vi "Lectura_TDMS.vi"() -> ()   [LabVIEW 2016]
panel:
  out "Waveform Graph 3":waveform(dbl)[](graph)
  out "Waveform Graph 2":waveform(dbl)[](graph)
  out "Waveform Graph":waveform(dbl)[](graph)
  in  "file path":path
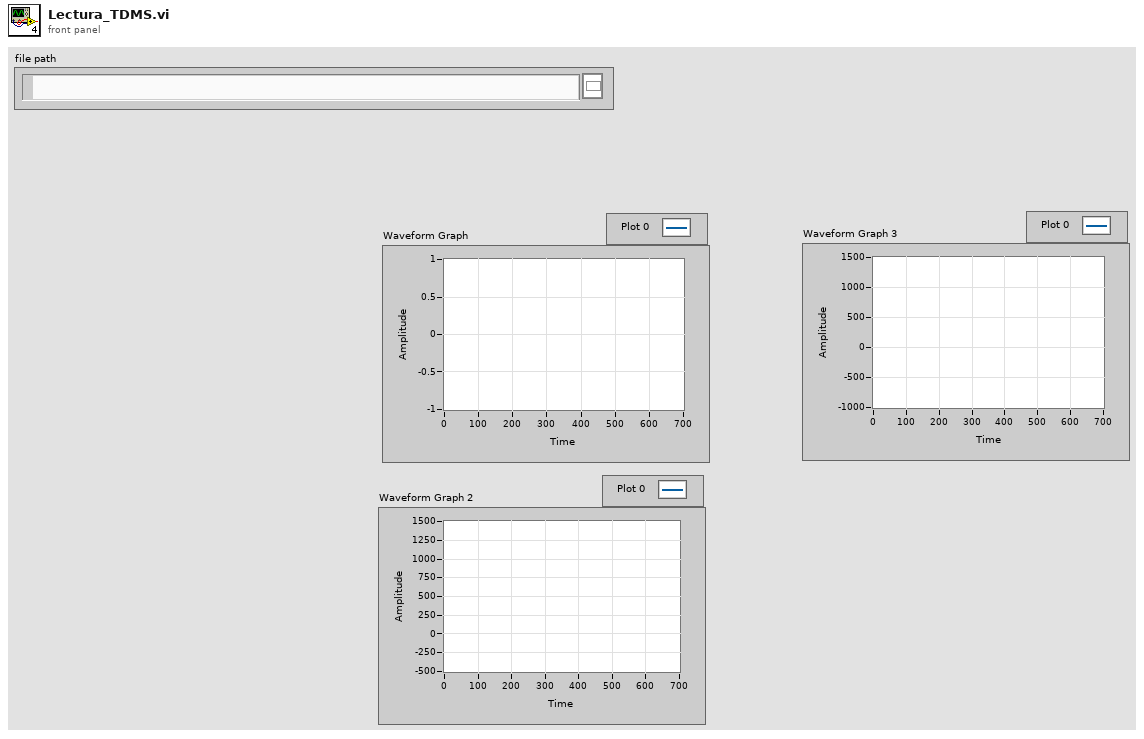
[diagram p1: front panel]
types:
  T1 = enum16{"open", "open or create", "create or replace", "create", "open (read-only)"}
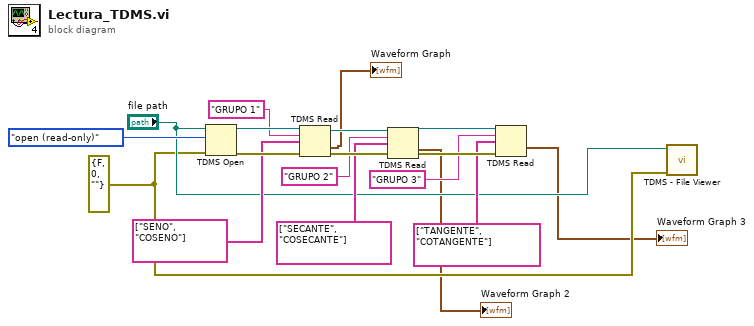
[diagram p0: block diagram]
diagram:
  w4 = errorcluster {"status"=FALSE, "code"=0, "source"=""} ("error in (no error)")
  n1 = TDMS Open(8:w4, 10:T1."open (read-only)" ("operation (0:open)"), 11:"file path") -> (0:w16:errorcluster, 3:w17:refnum<k34>)  [unwired: 4 in]
  n2 = TDMS Read(0:w17, 5:"GRUPO 1" ("group name in (Untitled)"), 7:string[] ["SENO", "COSENO"] ("channel name(s) in (Untitled)"), 11:w16) -> (4:w13:refnum<k34>, 10:→"Waveform Graph":waveform(dbl)[], 15:w12:errorcluster)  [unwired: 4 in, 3 out]
  n3 = TDMS Read(0:w13, 5:"GRUPO 2" ("group name in (Untitled)"), 7:string[] ["SECANTE", "COSECANTE"] ("channel name(s) in (Untitled)"), 11:w12) -> (4:w9:refnum<k34>, 10:→"Waveform Graph 2":waveform(dbl)[], 15:w8:errorcluster)  [unwired: 4 in, 3 out]
  n4 = TDMS Read(0:w9, 5:"GRUPO 3" ("group name in (Untitled)"), 7:string[] ["TANGENTE", "COTANGENTE"] ("channel name(s) in (Untitled)"), 11:w8) -> (10:→"Waveform Graph 3":waveform(dbl)[])  [unwired: 4 in, 5 out]
  n5 = call <vilib>:"TDMS - File Viewer.vi"("error in (no error)"=w4, "file path"="file path") -> ()  [unwired: 4 in, 2 out]
